vi "Init.vi"(8 "error in (no error)":errorcluster, 11 "uService Test in":refnum<class "test_us.lvclass">) -> (0 "error out":errorcluster, 3 "uService Test out":refnum<class "test_us.lvclass">)   [LabVIEW 2026, in "test_us.lvlib" / "test_us.lvclass"]
uses:
  test_us.lvclass
  C:/LabVIEW Code/TALOS/talos/Father of all uServices/Father of all uServices/Father of all uServices.lvclass
  Test uS Consumer case selector.ctl
  Ancestor/Ancestor/Infinite Message Selector.ctl
  Father of all uServices/Father of all uServices/Load Waveform Chart History - single plot.vi
  Ancestor/Ancestor/Ancestor.lvclass
  Father of all uServices/Father of all uServices/Father of all uServices.lvclass
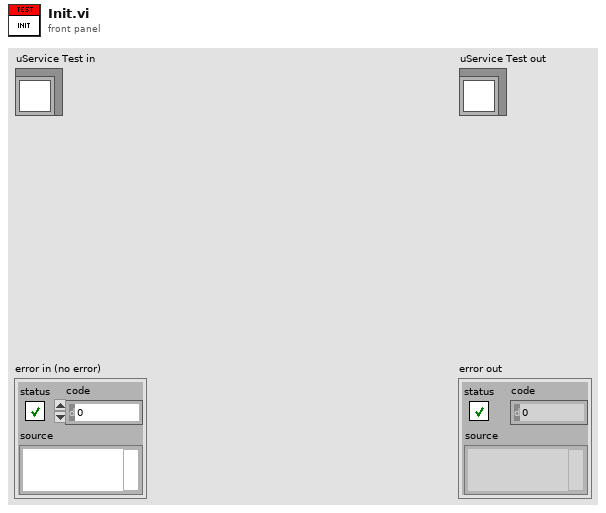
[diagram p1: front panel]
types:
  T1 = typedef "TALOS.lvlib/Ancestor.lvlib/Ancestor.lvclass/Infinite Message Selector.ctl" = enum16{"Start", "Stop", "Check", "Flush (Stop all)", "Init"}
  T2 = typedef "test_us.lvlib/test_us.lvclass/Test uS Consumer case selector.ctl" = enum16{"graph", "infinite", "Start infinite", "Check infinite", "Stop infinite", "Delayed message"}
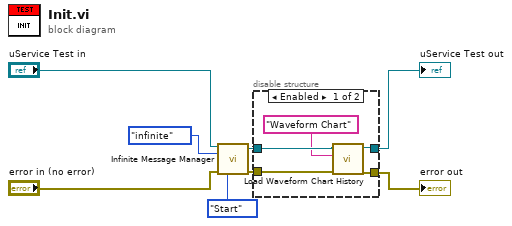
[diagram p0: block diagram]
diagram:
  n1 = call-dynamic "Infinite Message Manager.vi"("Father of all uServices in"="uService Test in", "Consumer Case Selector"=Test_uS_Consumer_case_selector."infinite" ("arsnars consumer case selector"), "error in (no error)"="error in (no error)", "Infinite Message Selector"=Infinite_Message_Selector."Start") -> ("Father of all uServices out"=w4:refnum<class "test_us.lvclass">, "error out"=w3:errorcluster)  [unwired: 9 in, 1 out]
  n2 = disable-structure shown="Enabled" {
    disable-tunnel: w4 -> [w13 w15]
    disable-tunnel: w3 -> [w10 w14]
    disable-tunnel: [w11 w14] -> w2
    disable-tunnel: [w12 w15] -> w1
    frame Enabled {
      n3 = call-poly "Load Waveform Chart History.vi"("error in (no error)"=w10, "Plot GUI label"="Waveform Chart", "Father of all uServices in"=w13) -> ("error out"=w11:errorcluster, "Father of all uServices out"=w12:refnum<class "test_us.lvclass">)  [unwired: 6 in, 1 out]
    }
    frame Disabled {
    }
  }
  "error out" <- w2
  "uService Test out" <- w1
